vi "Utility Write To Register.vi"(6 "Direct Action?":bool, 7 "Unit Address (1)":u8=1, 8 "error in (no error)":errorcluster, 9 "Data (0)":i16, 10 "Register Address (0)":u16, 11 "VISA resource name":refnum<visa-resource-name>) -> (0 "error out":errorcluster, 3 "VISA resource name out":refnum<visa-resource-name>)   [LabVIEW 2010]
doc: "This VI writes the value to the specified register of specified unit."
uses:
  MBDRV_Command Data.ctl
  MBDRV_Action.ctl
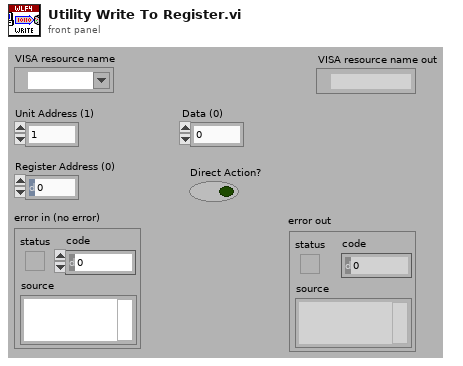
[diagram p1: front panel]
types:
  T1 = typedef "MBDRV_Command Data.ctl" = cluster{"Action":T2, "Com Port":string, "Register Address":u16, "Data To Write/Num To Read":i16}
  T2 = typedef "MBDRV_Action.ctl" = enum16{"Write", "Read"}
  T3 = enum16{"By The Number of Bytes", "Copy Of the Sent Message"}
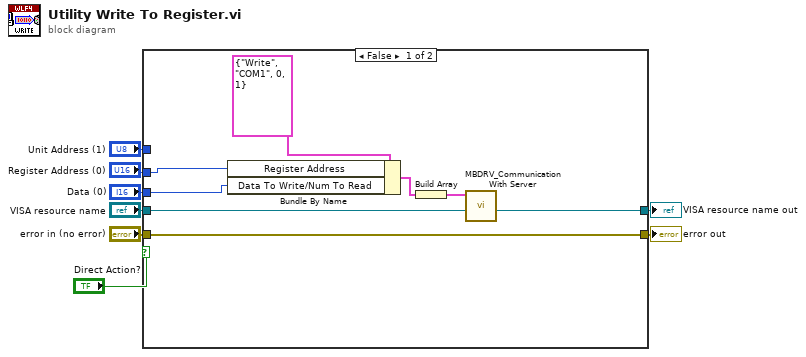
[diagram p0: block diagram]
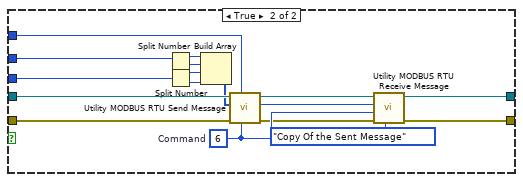
[diagram p2: hidden frame]
diagram:
  n1 = case shown="False" "Direct Action?" {
    tunnel: "VISA resource name" -> [w14 w32]
    tunnel: [w14 w31] -> w7
    tunnel: "Data (0)" -> [w10 w30]
    tunnel: [w15 w20] -> w5
    tunnel: "Unit Address (1)" -> [_ w19]
    tunnel: "Register Address (0)" -> [w9 w18]
    tunnel: "error in (no error)" -> [w15 w17]
    frame False {
      n2 = Bundle By Name(cluster=T1 {"Action"=enum."Write", "Com Port"="COM1", "Register Address"=0, "Data To Write/Num To Read"=1} ("Command"), "Register Address"=w9, "Data To Write/Num To Read"=w10) -> (w12:T1)
      n3 = Build Array(w12) -> (w11:T1[])
      n4 = call "MBDRV_Communication With Server.vi"("Write To PLC"=w11) -> ()  [unwired: 9 in, 2 out]
    }
    frame True {
      w28 = u8 6  # Command
      n5 = Split Number(x=w18) -> (hi(x)=w26:u8, lo(x)=w25:u8)
      n6 = Split Number(x=w30) -> (hi(x)=w24:u8, lo(x)=w23:u8)
      n7 = Build Array(w26, w25, w24, w23) -> (w27:u8[])
      n8 = call "Utility MODBUS RTU Send Message.vi"("Command (0)"=w28, "Unit Address (1)"=w19, "error in (no error)"=w17, "Message (empty array)"=w27, "VISA resource name"=w32) -> ("error out"=w16:errorcluster, "Length Of Sent MSG"=w22:u8, "VISA resource name out"=w29:refnum<visa-resource-name>)  [unwired: 4 in]
      n9 = call "Utility MODBUS RTU Receive Message.vi"("Receive Message Type (0: By The Number Of Bytes)"=T3."Copy Of the Sent Message" ("Receive Message Type"), "error in (no error)"=w16, "Sent Command (0)"=w28, "Length Of Sent MSG (0)"=w22, "VISA resource name"=w29) -> ("error out"=w20:errorcluster, "VISA resource name out"=w31:refnum<visa-resource-name>)  [unwired: 4 in, 1 out]
    }
  }
  "error out" <- w5
  "VISA resource name out" <- w7
